vi "Generate RAW Frame.vi"(8 "error in (no error)":errorcluster, 10 "Data to Send":T1 {"Identifier" format="%08x"}, 11 "connection info":T2) -> (0 "error out":errorcluster, 2 "Sent?":bool, 3 "connection info":T2)   [LabVIEW 2019, in "J1939 Addon Shared.lvlib"]
uses:
  <vilib>/NI/STM/TCP/TCP Connection Info.ctl
  <vilib>/NI/STM/SubVIs/MetaDataElement.ctl
  Support Libraries/J1939 Utilities/Types/CAN Outgoing Message Cluster.ctl
  J1939 Addon Shared.lvlib
  <vilib>/NI/NI VeriStand Addon Network Comm/Shared/NI VeriStand Addon Network Comm Shared.lvlib
  Support Libraries/J1939 Utilities/J1939 Utilities.lvlib
  <vilib>/NI/STM/NI STM.lvlib
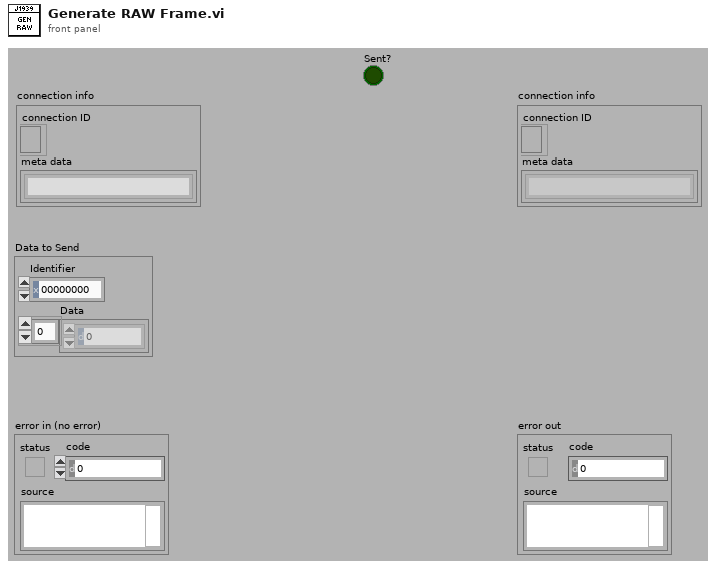
[diagram p1: front panel]
types:
  T1 = typedef "J1939 Utilities.lvlib/CAN Outgoing Message Cluster.ctl" = cluster{"Identifier":u32, "Data":u8[]}
  T2 = typedef "NI STM.lvlib/TCP Connection Info.ctl" = cluster{"connection ID":refnum<k5>, "meta data":T3[]}
  T3 = typedef "NI STM.lvlib/MetaDataElement.ctl" = string
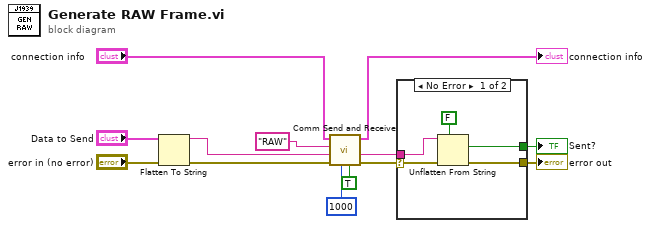
[diagram p0: block diagram]
diagram:
  n1 = Flatten To String(anything="Data to Send", error in (no error)="error in (no error)") -> (data string=w9:string, error out=w6:errorcluster)  [unwired: 2 in, 1 out]
  n2 = call <vilib>:"Comm Send and Receive.vi"("Resp Required?"=TRUE, "Timeout (ms)"=u32 1000 ("Timeout ms (5000)"), "error in (no error)"=w6, "Data"=w9, "Name"="RAW" ("Command"), "connection info"="connection info") -> ("error out"=w2:errorcluster, "Data"=w3:string, "connection info"=→"connection info":T2)  [unwired: 2 in, 1 out]
  n3 = case shown="No Error" w2 {
    selector: w2 -> [w16 w19]
    tunnel: [w15 w19] -> w4
    tunnel: w3 -> [w18 _]
    tunnel: [w14 _] -> w1
    frame No Error {
      n4 = Unflatten From String(type=FALSE, binary string=w18, error in (no error)=w16) -> (value=w14:bool, error out=w15:errorcluster)  [unwired: 2 in, 1 out]
    }
    frame Error {
    }
  }
  "error out" <- w4
  "Sent?" <- w1
